vi "Read2D.vi"(7 "Poll Time (ms)":u32=10, 8 "error in":errorcluster, 9 "Timeout (s)":dbl=5.0, 10 "Samps Read per Chan":i32, 11 "Task in":refnum<class "WaveformTask.lvclass">) -> (0 "error out":errorcluster, 1 "Samples Remaining":u32, 2 "Data":sgl[][](array[numeric]), 3 "Task out":refnum<class "WaveformTask.lvclass">)   [LabVIEW 2015, in "WaveformTask.lvclass"]
uses:
  WaveformTask.lvclass
  WaveformTask.lvclass/WaveformTask.ctl
  <vilib>/NI/cRIO Wfm/ErrorSelector.ctl
  <vilib>/rvi/errors/niLvFpgaAdjustHostInterfaceError.vi
  <vilib>/Utility/error.llb/Error Cluster From Error Code.vi
  DataFIFOs.ctl
  <vilib>/rvi/interface/nirviMethod/nirviMethod.xnode
  <vilib>/FPGAPlugInAG/Dynamic/niLvFpga_ReadFifo_Dynamic.vi
  <vilib>/rvi/errors/niLvFpgaMergeErrorWithErrorCode.vi
  <vilib>/NI/cRIO Wfm/cRIO Wfm.lvlib
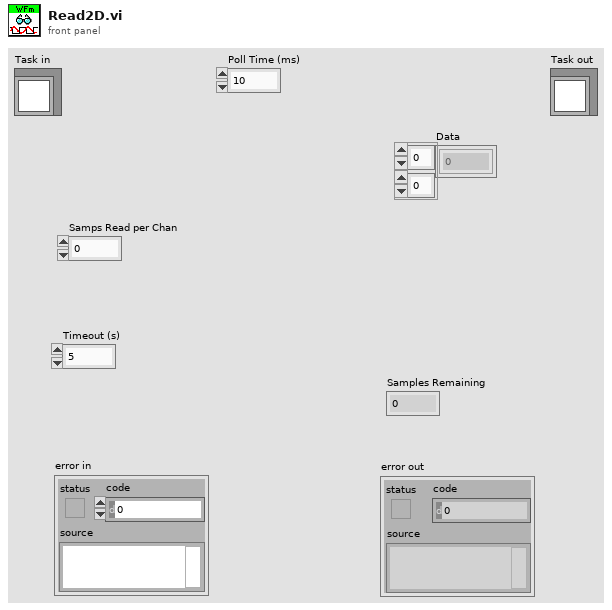
[diagram p1: front panel]
types:
  T1 = typedef "WaveformTask.lvclass/DataFIFOs.ctl" = refnum<k20>
  T2 = typedef "cRIO Wfm.lvlib/ErrorSelector.ctl" = enum16{"Read Timeout", "Module Underflow", "DMA Overflow", "Chan Count", "Run Timeout", "Start Timeout", "Stop Timeout"}
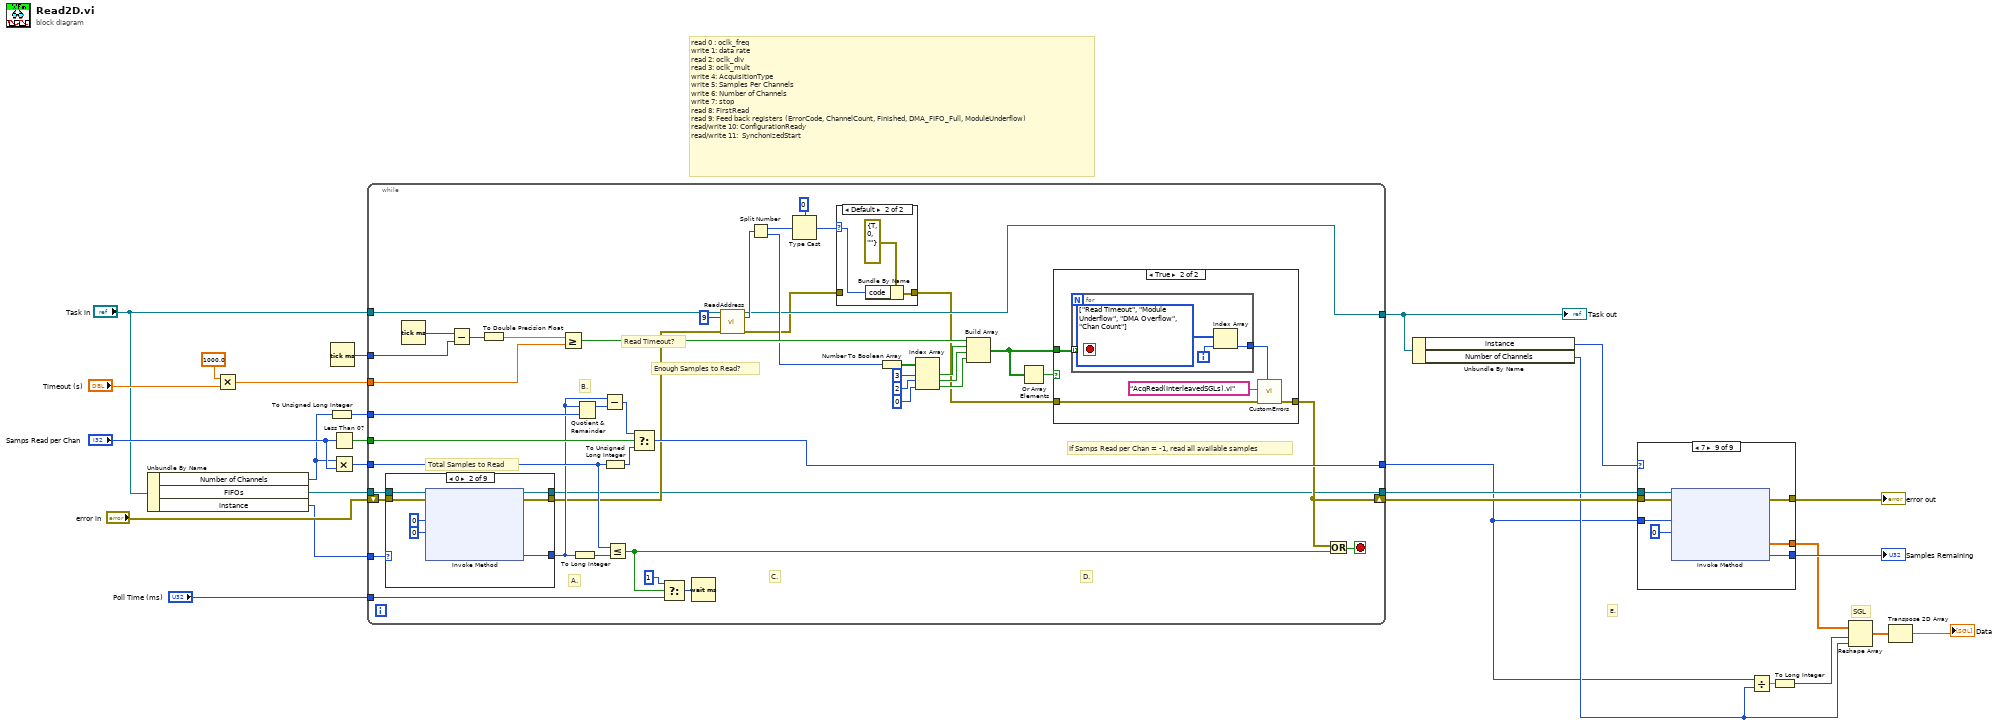
[diagram p0: block diagram]
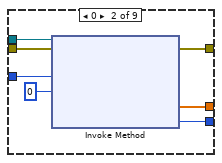
[diagram p3: hidden frame]
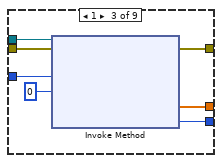
[diagram p4: hidden frame]
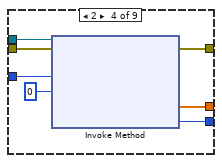
[diagram p5: hidden frame]
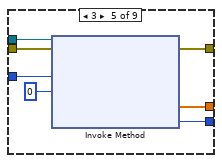
[diagram p6: hidden frame]
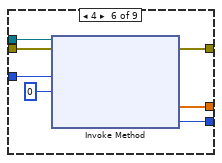
[diagram p7: hidden frame]
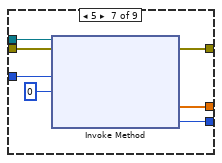
[diagram p8: hidden frame]
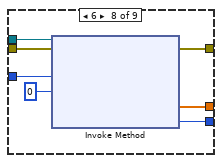
[diagram p9: hidden frame]
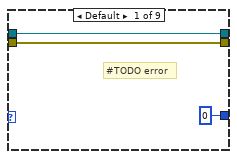
[diagram p11: hidden frame]
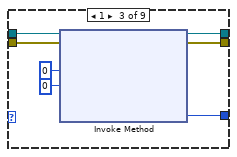
[diagram p12: hidden frame]
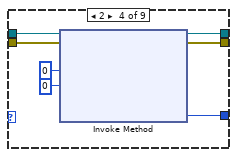
[diagram p13: hidden frame]
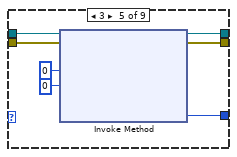
[diagram p14: hidden frame]
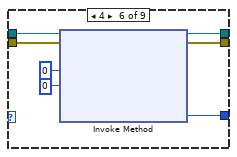
[diagram p15: hidden frame]
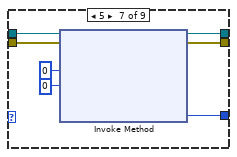
[diagram p16: hidden frame]
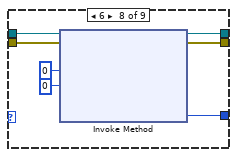
[diagram p17: hidden frame]
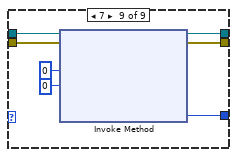
[diagram p18: hidden frame]
diagram:
  # "SGL"
  # "read 0 : oclk_freq\nwrite 1: data rate\nread 2: oclk_div\nread 3: oclk_mult\nwrite 4: AcquisitionType\nwrite 5: Samples Per Channels\nwrite 6: Number of Channels\nwrite 7: stop\nread 8: FirstRead\nread 9: Feed back registers (ErrorCode, ChannelCount, Finished, DMA_FIFO_Full, ModuleUnderflow)\nread/write 10: ConfigurationReady\nread/write 11:  SynchonizedStart"
  # "E."
  n1 = Unbundle By Name("Task in") -> ("Number of Channels"=w12:i32, "FIFOs"=w13:T1, "instance"=w10:u8)
  n2 = Multiply(x=1000.0 ("y"), y="Timeout (s)") -> (x*y=w24:dbl)
  n3 = To Unsigned Long Integer(number=w12) -> (unsigned 32bit integer=w19:u32)
  n4 = Tick Count (ms)() -> (millisecond timer value=w26:u32)
  n5 = Less Than 0?(x="Samps Read per Chan") -> (x < 0?=w21:bool)
  n6 = Multiply(x=w12, y="Samps Read per Chan") -> (x*y=w20:i32)
  n7 = while {
    tunnel: [w33] -> w22
    tunnel: w13 -> [w67]
    tunnel: w26 -> [w69]
    tunnel: w24 -> [w68]
    tunnel: "Poll Time (ms)" -> [w61]
    tunnel: [w54] -> w2
    tunnel: w20 -> [w56]
    tunnel: w21 -> [w57]
    tunnel: w19 -> [w58]
    shift-right: [w48] -> w23
    shift-left: "error in" -> [w66]
    tunnel: "Task in" -> [w47]
    tunnel: [w32] -> w9
    tunnel: w10 -> [w31]
    stop <- w72 stop-if-true
    # "A."
    # "D."
    # "C."
    # "B."
    # "If Samps Read per Chan = -1, read all available samples"
    # "Read Timeout?"
    # "Total Samples to Read"
    # "Enough Samples to Read?"
    n8 = case shown="0" w31 {
      tunnel: w67 -> [w79 w86 w93 w100 w107 w114 w121 w128 w135]
      tunnel: w66 -> [w78 w85 w92 w99 w106 w113 w120 w127 w134]
      tunnel: [u32 0 ("Elements Remaining") w82 w89 w96 w103 w110 w117 w124 w131] -> w51
      tunnel: [w78 w81 w88 w95 w102 w109 w116 w123 w130] -> w40
      tunnel: [w79 w80 w87 w94 w101 w108 w115 w122 w129] -> w33
      frame Default {
        # "#TODO error"
      }
      frame 0 {
        n9 = xnode "Invoke Method"("FPGA VI Reference In"=w86, "error in"=w85, "Number of Elements"=u32 0, "Timeout (ms)"=0) -> ("FPGA VI Reference Out"=w80:T1, "error out"=w81:errorcluster, "Elements Remaining"=w82:u32)  [unwired: 1 out]
      }
      frame 1 {
        n10 = xnode "Invoke Method"("FPGA VI Reference In"=w93, "error in"=w92, "Number of Elements"=u32 0, "Timeout (ms)"=0) -> ("FPGA VI Reference Out"=w87:T1, "error out"=w88:errorcluster, "Elements Remaining"=w89:u32)  [unwired: 1 out]
      }
      frame 2 {
        n11 = xnode "Invoke Method"("FPGA VI Reference In"=w100, "error in"=w99, "Number of Elements"=u32 0, "Timeout (ms)"=0) -> ("FPGA VI Reference Out"=w94:T1, "error out"=w95:errorcluster, "Elements Remaining"=w96:u32)  [unwired: 1 out]
      }
      frame 3 {
        n12 = xnode "Invoke Method"("FPGA VI Reference In"=w107, "error in"=w106, "Number of Elements"=u32 0, "Timeout (ms)"=0) -> ("FPGA VI Reference Out"=w101:T1, "error out"=w102:errorcluster, "Elements Remaining"=w103:u32)  [unwired: 1 out]
      }
      frame 4 {
        n13 = xnode "Invoke Method"("FPGA VI Reference In"=w114, "error in"=w113, "Number of Elements"=u32 0, "Timeout (ms)"=0) -> ("FPGA VI Reference Out"=w108:T1, "error out"=w109:errorcluster, "Elements Remaining"=w110:u32)  [unwired: 1 out]
      }
      frame 5 {
        n14 = xnode "Invoke Method"("FPGA VI Reference In"=w121, "error in"=w120, "Number of Elements"=u32 0, "Timeout (ms)"=0) -> ("FPGA VI Reference Out"=w115:T1, "error out"=w116:errorcluster, "Elements Remaining"=w117:u32)  [unwired: 1 out]
      }
      frame 6 {
        n15 = xnode "Invoke Method"("FPGA VI Reference In"=w128, "error in"=w127, "Number of Elements"=u32 0, "Timeout (ms)"=0) -> ("FPGA VI Reference Out"=w122:T1, "error out"=w123:errorcluster, "Elements Remaining"=w124:u32)  [unwired: 1 out]
      }
      frame 7 {
        n16 = xnode "Invoke Method"("FPGA VI Reference In"=w135, "error in"=w134, "Number of Elements"=u32 0, "Timeout (ms)"=0) -> ("FPGA VI Reference Out"=w129:T1, "error out"=w130:errorcluster, "Elements Remaining"=w131:u32)  [unwired: 1 out]
      }
    }
    n17 = Tick Count (ms)() -> (millisecond timer value=w65:u32)
    n18 = Subtract(x=w65, y=w69) -> (x-y=w71:u32)
    n19 = To Double Precision Float(number=w71) -> (double precision float=w70:dbl)
    n20 = Greater Or Equal?(x=w70, y=w68) -> (x >= y?=w64:bool)
    n21 = To Long Integer(number=w51) -> (32bit integer=w59:i32)
    n22 = Quotient & Remainder(x=w51, y=w58) -> (x-y*floor(x/y)=w53:u32)  [unwired: 1 out]
    n23 = Subtract(x=w51, y=w53) -> (x-y=w52:u32)
    n24 = To Unsigned Long Integer(number=w56) -> (unsigned 32bit integer=w55:u32)
    n25 = Less Or Equal?(x=w56, y=w59) -> (x <= y?=w62:bool)
    n26 = Select(t=w52, s=w57, f=w55) -> (s? t:f=w54:u32)
    n27 = Select(t=u32 1, s=w62, f=w61) -> (s? t:f=w63:u32)
    n28 = Wait (ms)(milliseconds to wait=w63) -> ()  [unwired: 1 out]
    n29 = call "ReadAddress.vi"("Task in"=w47, "address"=u64 9, "error in (no error)"=w40) -> ("Task out"=w32:refnum<class "WaveformTask.lvclass">, "data"=w45:u64, "error out"=w29:errorcluster)  [unwired: 10 in]
    n30 = Split Number(x=w45) -> (hi(x)=w44:u32, lo(x)=w42:u32)
    n31 = Type Cast(type=0, x=w44) -> (*(type *) &x=w30:i32)
    n32 = case shown="Default" w30 {
      selector: w30 -> [_ w75]
      tunnel: w29 -> [w73 _]
      tunnel: [w73 w74] -> w28
      frame 0 {
      }
      frame Default {
        n33 = Bundle By Name(cluster=errorcluster {"status"=TRUE, "code"=0, "source"=""} ("error out"), "code"=w75) -> (w74:errorcluster)
      }
    }
    n34 = Number To Boolean Array(number=w42) -> (Boolean array=w41:bool[])
    n35 = Index Array(array=w41, index #1=3 ("index"), index #2=2 ("index"), index #3=0 ("index")) -> (element #1=w36:bool, element #2=w35:bool, element #3=w34:bool)
    n36 = Build Array(w64, w36, w35, w34) -> (w49:bool[])
    n37 = Or Array Elements(Boolean array=w49) -> (logical OR=w50:bool)
    n38 = case shown="True" w50 {
      tunnel: [w136 w140] -> w48
      tunnel: w28 -> [w136 w141]
      tunnel: w49 -> [_ w139]
      frame False {
      }
      frame True {
        n39 = for {
          tunnel: w139 -> [w145] mode=indexing
          tunnel: [w142] -> w138
          i -> [w143]
          stop <- w145 stop-if-true
          w144 = T2[] [enum."Read Timeout", enum."Module Underflow", enum."DMA Overflow", enum."Chan Count"] items=["Read Timeout", "Module Underflow", "DMA Overflow", "Chan Count", "Run Timeout", "Start Timeout", "Stop Timeout"]
          n40 = Index Array(array=w144, index=w143) -> (element=w142:T2)
        }
        n41 = call <vilib>:"CustomErrors.vi"("Error Selector"=w138, "error in"=w141, "Calling VI"="AcqRead(InterleavedSGLs).vi") -> ("error out"=w140:errorcluster)  [unwired: 8 in]
      }
    }
    n42 = Or(x=w48, y=w62) -> (x .or. y?=w72:bool)
  }
  "Task out" <- w9
  n43 = Unbundle By Name(w9) -> ("instance"=w8:u8, "Number of Channels"=w3:i32)
  n44 = case shown="7" w8 {
    tunnel: [w146 w153 w160 w167 w174 w181 w188 w195 w202] -> w27
    tunnel: w23 -> [w146 w152 w159 w166 w173 w180 w187 w194 w201]
    tunnel: w22 -> [_ w151 w158 w165 w172 w179 w186 w193 w200]
    tunnel: w2 -> [_ w150 w157 w164 w171 w178 w185 w192 w199]
    tunnel: [_ w148 w155 w162 w169 w176 w183 w190 w197] -> w4
    tunnel: [_ w147 w154 w161 w168 w175 w182 w189 w196] -> w14
    frame Default {
      # "#TODO Error"
    }
    frame 0 {
      n45 = xnode "Invoke Method"("FPGA VI Reference In"=w151, "error in"=w152, "Number of Elements"=w150, "Timeout (ms)"=0) -> ("error out"=w153:errorcluster, "Data"=w148:sgl[], "Elements Remaining"=w147:u32)  [unwired: 1 out]
    }
    frame 1 {
      n46 = xnode "Invoke Method"("FPGA VI Reference In"=w158, "error in"=w159, "Number of Elements"=w157, "Timeout (ms)"=0) -> ("error out"=w160:errorcluster, "Data"=w155:sgl[], "Elements Remaining"=w154:u32)  [unwired: 1 out]
    }
    frame 2 {
      n47 = xnode "Invoke Method"("FPGA VI Reference In"=w165, "error in"=w166, "Number of Elements"=w164, "Timeout (ms)"=0) -> ("error out"=w167:errorcluster, "Data"=w162:sgl[], "Elements Remaining"=w161:u32)  [unwired: 1 out]
    }
    frame 3 {
      n48 = xnode "Invoke Method"("FPGA VI Reference In"=w172, "error in"=w173, "Number of Elements"=w171, "Timeout (ms)"=0) -> ("error out"=w174:errorcluster, "Data"=w169:sgl[], "Elements Remaining"=w168:u32)  [unwired: 1 out]
    }
    frame 4 {
      n49 = xnode "Invoke Method"("FPGA VI Reference In"=w179, "error in"=w180, "Number of Elements"=w178, "Timeout (ms)"=0) -> ("error out"=w181:errorcluster, "Data"=w176:sgl[], "Elements Remaining"=w175:u32)  [unwired: 1 out]
    }
    frame 5 {
      n50 = xnode "Invoke Method"("FPGA VI Reference In"=w186, "error in"=w187, "Number of Elements"=w185, "Timeout (ms)"=0) -> ("error out"=w188:errorcluster, "Data"=w183:sgl[], "Elements Remaining"=w182:u32)  [unwired: 1 out]
    }
    frame 6 {
      n51 = xnode "Invoke Method"("FPGA VI Reference In"=w193, "error in"=w194, "Number of Elements"=w192, "Timeout (ms)"=0) -> ("error out"=w195:errorcluster, "Data"=w190:sgl[], "Elements Remaining"=w189:u32)  [unwired: 1 out]
    }
    frame 7 {
      n52 = xnode "Invoke Method"("FPGA VI Reference In"=w200, "error in"=w201, "Number of Elements"=w199, "Timeout (ms)"=0) -> ("error out"=w202:errorcluster, "Data"=w197:sgl[], "Elements Remaining"=w196:u32)  [unwired: 1 out]
    }
  }
  "error out" <- w27
  "Samples Remaining" <- w14
  n53 = Divide(x=w2, y=w3) -> (x/y=w6:dbl)
  n54 = To Long Integer(number=w6) -> (32bit integer=w5:i32)
  n55 = Reshape Array(w4, w5, w3) -> (w7:sgl[][])
  n56 = Transpose 2D Array(2D array=w7) -> (transposed array=→"Data":sgl[][])
